vi "CalculateAbsWind.vi"(11 "NotifierReff":T1) -> ()   [LabVIEW 2013]
doc: "THIS VI IS UNTESTED AND NEEDS TO BE CALIBRATED ON THE WATER.\n\nThe point of this VI is to take in data from the sensors and calculates absolute wind. It then writes that to the AbsWindDirection notifier.\n\nEric Schneider, March 2014"
uses:
  Data/TypeDefs/Notifiers.ctl
  Data/TypeDefs/UTM Location.ctl
  Data/TypeDefs/Sail Set Suggestions.ctl
  Data/TypeDefs/Rudder Set Suggestions.ctl
  Data/TypeDefs/OverrideInformation.ctl
  Data/TypeDefs/OverrideMode.ctl
  Data/TypeDefs/MotorSetup.ctl
  Data/TypeDefs/DynamixelSetupInfo.ctl
  Data/TypeDefs/AirmarStatus.ctl
  Data/TypeDefs/HardwareOnline.ctl
  Data/TypeDefs/DynamixelCycleTracker.ctl
  Utilities/Math/Vectors/CartesianVector/CartesianVector.lvclass
  Utilities/Math/Angles/Angle/Angle.lvclass
panel:
  out "AbsWindDirection":dbl
  in  "Wind Speed":dbl
  in  "RelWindDirection":dbl
  in  "Boat Speed":dbl
  in  "Debug by hand?":bool
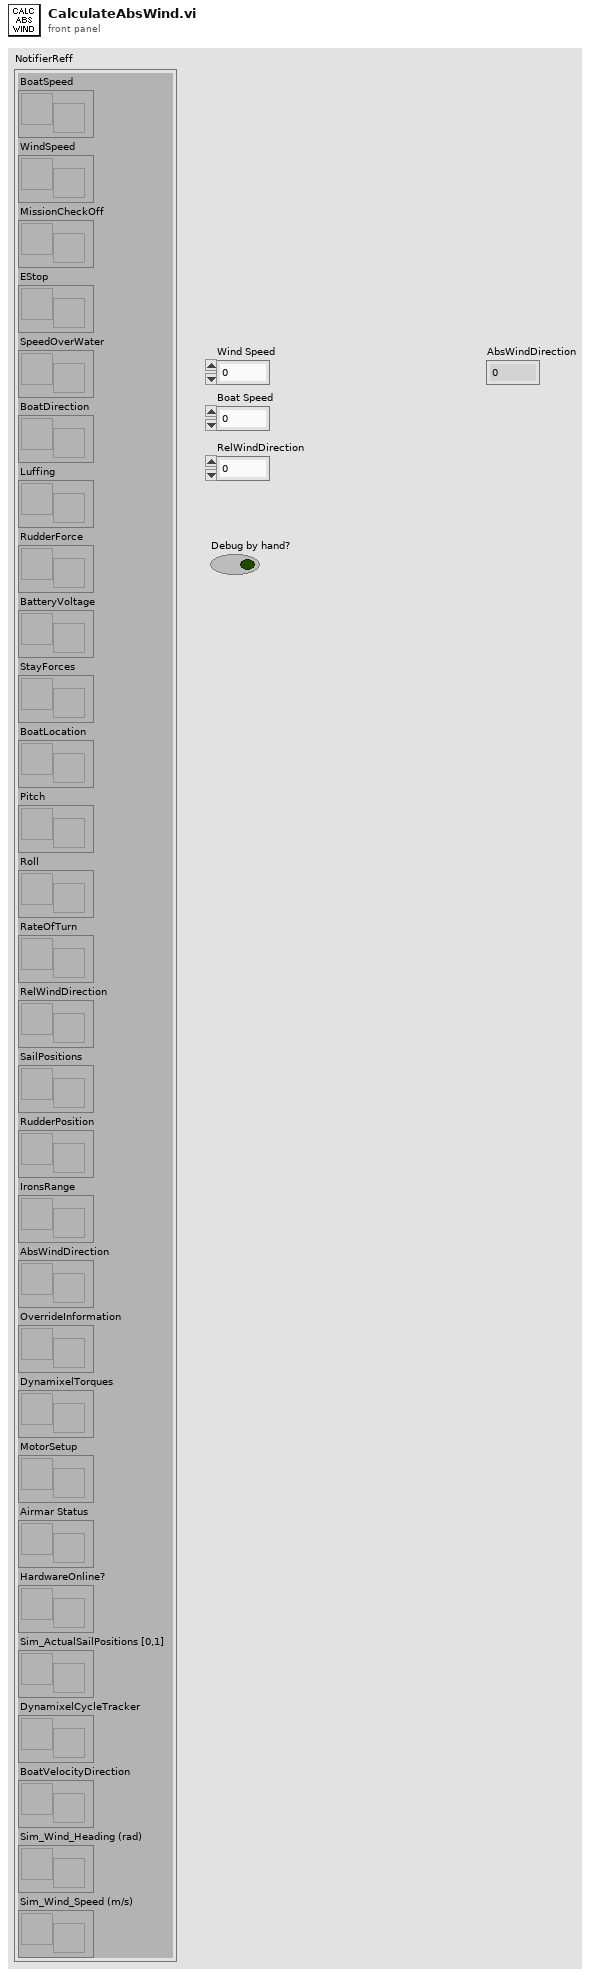
[diagram p1: front panel]
types:
  T1 = typedef "Notifiers.ctl" = cluster{"BoatSpeed":refnum<notifier>, "WindSpeed":refnum<notifier>, "MissionCheckOff":refnum<notifier>, "EStop":refnum<notifier>, "SpeedOverWater":refnum<notifier>, "BoatDirection":refnum<notifier>, "Luffing":refnum<notifier>, "RudderForce":refnum<notifier>, "BatteryVoltage":refnum<notifier>, "StayForces":refnum<notifier>, "BoatLocation":refnum<notifier>, "Pitch":refnum<notifier>, "Roll":refnum<notifier>, "RateOfTurn":refnum<notifier>, "RelWindDirection":refnum<notifier>, "SailPositions":refnum<notifier>, "RudderPosition":refnum<notifier>, "IronsRange":refnum<notifier>, "AbsWindDirection":refnum<notifier>, "OverrideInformation":refnum<notifier>, "DynamixelTorques":refnum<notifier>, "MotorSetup":refnum<notifier>, "Airmar Status":refnum<notifier>, "HardwareOnline?":refnum<notifier>, "Sim_ActualSailPositions [0,1]":refnum<notifier>, "DynamixelCycleTracker":refnum<notifier>, "BoatVelocityDirection":refnum<notifier>, "Sim_Wind_Heading (rad)":refnum<notifier>, "Sim_Wind_Speed (m/s)":refnum<notifier>}
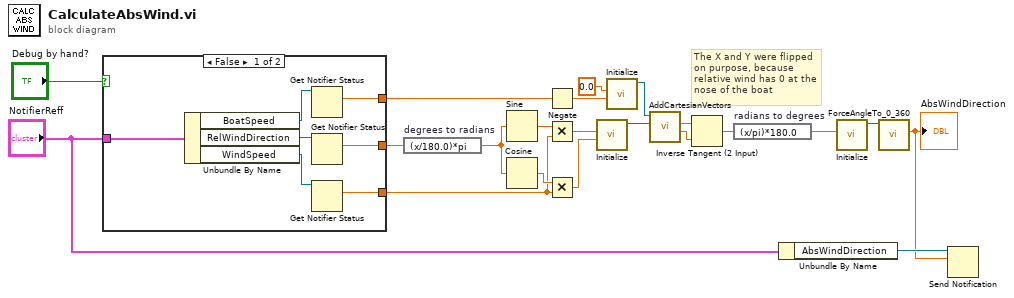
[diagram p0: block diagram]
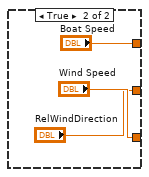
[diagram p2: hidden frame]
diagram:
  # "The X and Y were flipped on purpose, because relative wind has 0 at the nose of the boat"
  n1 = case shown="False" "Debug by hand?" {
    tunnel: [w27 "RelWindDirection"] -> w21
    tunnel: [w25 "Wind Speed"] -> w17
    tunnel: [w23 "Boat Speed"] -> w14
    tunnel: "NotifierReff" -> [w22 _]
    frame False {
      n2 = Unbundle By Name(w22) -> ("BoatSpeed"=w24:refnum<notifier>, "RelWindDirection"=w28:refnum<notifier>, "WindSpeed"=w26:refnum<notifier>)
      n3 = Get Notifier Status(notifier=w24) -> (current notification=w23:dbl)  [unwired: 1 in, 4 out]
      n4 = Get Notifier Status(notifier=w28) -> (current notification=w27:dbl)  [unwired: 1 in, 4 out]
      n5 = Get Notifier Status(notifier=w26) -> (current notification=w25:dbl)  [unwired: 1 in, 4 out]
    }
    frame True {
    }
  }
  n6 = expression code="(x/180.0)*pi" "degrees to radians"(w21) -> (w20:dbl)
  n7 = Sine(x=w20) -> (sin(x)=w19:dbl)
  n8 = Cosine(x=w20) -> (cos(x)=w18:dbl)
  n9 = Negate(x=w14) -> (-x=w13:dbl)
  n10 = Multiply(x=w19, y=w17) -> (x*y=w16:dbl)
  n11 = Multiply(x=w18, y=w17) -> (x*y=w15:dbl)
  n12 = call "Initialize.vi"("Y (North)"=w15, "X (East)"=w16) -> ("CartesianVector out"=w10:refnum<class "CartesianVector.lvclass">)  [unwired: 8 in, 1 out]
  n13 = call "Initialize.vi"("Y (North)"=w13, "X (East)"=0.0) -> ("CartesianVector out"=w11:refnum<class "CartesianVector.lvclass">)  [unwired: 8 in, 1 out]
  n14 = call "AddCartesianVectors.vi"("CartesianVector in B"=w10, "CartesianVector in A"=w11) -> ("Y (North)"=w6:dbl, "X (East)"=w7:dbl)  [unwired: 6 in, 2 out]
  n15 = Inverse Tangent (2 Input)(1:w6, 2:w7) -> (0:w8:dbl)
  n16 = expression code="(x/pi)*180.0" "radians to degrees"(w8) -> (w5:dbl)
  n17 = Unbundle By Name("NotifierReff") -> ("AbsWindDirection"=w2:refnum<notifier>)
  n18 = call "Initialize.vi"("Input Angle (Deg.)"=w5) -> ("Angle out"=w4:refnum<class "Angle.lvclass">)  [unwired: 9 in, 1 out]
  n19 = call "ForceAngleTo_0_360.vi"("Angle in"=w4) -> ("Relative Angle"=w1:dbl)  [unwired: 9 in, 1 out]
  "AbsWindDirection" <- w1
  n20 = Send Notification(notification=w1, notifier=w2) -> ()  [unwired: 1 in, 2 out]
